vi "HOST_feedbacktest_datamonitoring_AAoptAOD_8-17-23.vi"() -> ()   [LabVIEW 2020]
uses:
  <vilib>/rvi/interface/nirviMethod/nirviMethod.xnode
  <vilib>/rvi/errors/niLvFpgaMergeErrorWithErrorCode.vi
  <instrlib>/_niInstr/Streaming/v1/Host/niInstr Streaming v1 Host.lvlib
  <vilib>/rvi/interface/nirviReadWriteControl/nirviReadWriteControl.xnode
  <vilib>/rvi/interface/nirviCloseFPGA/nirviCloseFPGA.xnode
  <vilib>/rvi/interface/nirviOpenFPGA/nirviOpenFPGA.xnode
  <vilib>/rvi/interface/Simulation/niFpgaSimulationCallBeginRW.vi
  <vilib>/rvi/errors/niLvFpgaAdjustHostInterfaceError.vi
  NiFpgaLv.dll
  <vilib>/Utility/error.llb/Error Cluster From Error Code.vi
  <vilib>/Utility/file.llb/Write Delimited Spreadsheet (string).vi
  <instrlib>/_niInstr/Streaming/v1/Host/Public/Start Finite Stream.vi
  <instrlib>/_niInstr/Streaming/v1/Host/Public/Wait for Stream.vi
  <vilib>/FPGAPlugInAG/Dynamic/niLvFpga_WriteFifo_Dynamic.vi
  <vilib>/FPGAPlugInAG/Dynamic/niLvFpga_Close_Dynamic.vi
  <vilib>/FPGAPlugInAG/Dynamic/niLvFpga_ReadFifo_Dynamic.vi
  <instrlib>/_niInstr/Streaming/v1/Host/Public/Start Continuous Stream.vi
  <vilib>/FPGAPlugInAG/Dynamic/niLvFpga_ConfigureFifo_Dynamic.vi
  <vilib>/FPGAPlugInAG/Dynamic/niLvFpga_StartFifo_Dynamic.vi
  FPGA Bitfiles/rfsignal_FPGATarget_feedbacktestdata_LKc-S6OmDz4.lvbitx
  <vilib>/FPGAPlugInAG/PXIe-7972R/niLvFpga_Open_PXIe-7972R.vi
  <vilib>/rvi/interface/common/dynamic/niFpgaDynamicAddResources.vi
  <vilib>/userdefined/Silver/nirio_resource_slv.ctl
  Controls/Clock Select.ctl
  PID/Typedef/niFpgaPID_ManualControl.ctl
  PID/Typedef/niFpgaPID_PIDGains.ctl
  PID/Typedef/niFpgaPID_OutputRange.ctl
  PID/Typedef/niFpgaPID_SetpointWeightings.ctl
  PID/Typedef/niFpgaPID_PIDActions.ctl
panel:
  out "actions":T1
  out "error":sgl
  out "output":sgl
  out "error 2":sgl
  out "error 3":sgl
  out "output 3":sgl
  out "actions 3":T1
  out "output 2":sgl
  out "actions 2":T1
  in  "Gains Z":T2[](array[typedef]) {"filter coefficient" min=0 max=1; "proportional gain" step=0.125}
  in  "setpoint weighting 3":T3={"proportional weighting (1)"=1.0, "derivative weighting (0)"=0.0} {"derivative weighting (0)" min=0 max=1; "proportional weighting (1)" min=0 max=1}
  in  "output range 3":T4={"output high (Inf)"=inf, "output low (-Inf)"=-inf}
  in  "manual control 3":T5
  in  "reset? (F) 3":bool
  in  "setpoint weighting 2":T3={"proportional weighting (1)"=1.0, "derivative weighting (0)"=0.0} {"derivative weighting (0)" min=0 max=1; "proportional weighting (1)" min=0 max=1}
  in  "output range 2":T4={"output high (Inf)"=inf, "output low (-Inf)"=-inf}
  in  "gains 2":T2 {"filter coefficient" min=0 max=1; "proportional gain" step=0.125}
  in  "manual control 2":T5
  in  "reset? (F) 2":bool
  in  "Feedback scaling z":fxp<+,16,4>
  in  "Feedback scaling x/y":fxp<+,16,4>
  in  "Apply feedback":bool
  in  "Data Trigger Level (V)":dbl
  in  "Record Size":u16=1024
  out "AI":waveform(dbl)[](graph)
  in  "Data Trigger When":enum8{"Trigger Above", "Trigger Below"}(ring)
  in  "Trigger Type":enum8{"Immediate", "Data Trigger", "TRIG input"}(ring)
  in  "Direction switch":bool
  in  "Step gain values":dbl
  in  "?":bool
  in  "% of max CH 1":dbl=85.0
  in  "% of max CH 0":dbl=85.0
  in  "setpoint weighting":T3={"proportional weighting (1)"=1.0, "derivative weighting (0)"=0.0} {"derivative weighting (0)" min=0 max=1; "proportional weighting (1)" min=0 max=1}
  in  "output range":T4={"output high (Inf)"=inf, "output low (-Inf)"=-inf}
  in  "gains":T2 {"filter coefficient" min=0 max=1; "proportional gain" step=0.125}
  in  "manual control":T5
  in  "reset? (F)":bool
  in  "write time ch0":bool
  in  "Record time for power sweep CH0":bool
  in  "Record time for power sweep CH1":bool
  in  "write time ch1":bool
  in  "save path for power calibration (dialog if empty)":path
  out "time check":u16=16
  in  "Cycles per step":u16=30
  in  "Gain Scan Endpoint (CH1)":dbl[](array[numeric])=[100.0, 100.0, 100.0, 100.0, 100.0, 100.0, 100.0, 100.0, 100.0, 100.0, 100.0, 100.0, 100.0, 100.0, 100.0, 100.0, 100.0, 100.0, 100.0, 100.0, 100.0, 100.0, 100.0, 100.0, 100.0, 100.0, 100.0, 100.0, 100.0, 100.0, 100.0, 100.0, 100.0, 100.0, 100.0, 100.0]
  in  "Gain Scan Endpoint (CH0)":dbl[](array[numeric])=[100.0, 100.0, 100.0, 100.0, 100.0, 100.0, 100.0, 100.0, 100.0, 100.0, 100.0, 100.0, 100.0, 100.0, 100.0, 100.0, 100.0, 100.0, 100.0, 100.0, 100.0, 100.0, 100.0, 100.0, 100.0, 100.0, 100.0, 100.0, 100.0, 100.0, 100.0, 100.0, 100.0, 100.0, 100.0, 100.0]
  in  "Scan End Setpoint (CH1)":dbl[](array[numeric])=[23.0, 24.0, 25.0, 26.0, 27.0, 28.0, 23.0, 24.0, 25.0, 26.0, 27.0, 28.0, 23.0, 24.0, 25.0, 26.0, 27.0, 28.0, 23.0, 24.0, 25.0, 26.0, 27.0, 28.0, 23.0, 24.0, 25.0, 26.0, 27.0, 28.0, 23.0, 24.0, 25.0, 26.0, 27.0, 28.0] format="%#_10f"
  in  "Scan CH1":bool
  in  "Scan CH0":bool
  in  "Fq Scan Endpoint (CH0)":dbl[](array[numeric])=[23.0, 23.0, 23.0, 23.0, 23.0, 23.0, 24.0, 24.0, 24.0, 24.0, 24.0, 24.0, 25.0, 25.0, 25.0, 25.0, 25.0, 25.0, 26.0, 26.0, 26.0, 26.0, 26.0, 26.0, 27.0, 27.0, 27.0, 27.0, 27.0, 27.0, 28.0, 28.0, 28.0, 28.0, 28.0, 28.0] format="%#_10f"
  in  "Refresh Integral":bool
  in  "Amp mod on/off":bool[](array[boolean])=[FALSE, FALSE, FALSE, FALSE, FALSE, FALSE, FALSE, FALSE, FALSE]
  in  "Mod Amp (%)":fxp<+,16,1>[](array[numeric])=[1.0, 1.0, 1.0, 1.0, 1.0, 1.0, 1.0, 1.0, 1.0]
  in  "Mod Fq (Hz) 3":dbl[](array[numeric])=[1.0, 1.0, 1.0, 1.0, 1.0, 1.0, 1.0, 1.0, 1.0] format="%#5.5f"
  in  "Wave 2 mod on/off":bool[](array[boolean])=[FALSE, FALSE, FALSE, FALSE, FALSE, FALSE, FALSE, FALSE, FALSE]
  in  "Mod strength (Hz) 2":dbl[](array[numeric])=[100000.0, 100000.0, 100000.0, 100000.0, 100000.0, 100000.0, 100000.0, 100000.0, 100000.0] format="%#_6p"
  in  "Mod Fq (Hz) 2":dbl[](array[numeric])=[1.0, 1.0, 1.0, 1.0, 1.0, 1.0, 1.0, 1.0, 1.0] format="%#5.5f"
  in  "Wave 1 mod on/off":bool[](array[boolean])=[FALSE, FALSE, FALSE, FALSE, FALSE, FALSE, FALSE, FALSE, FALSE]
  in  "Mod strength (Hz)":dbl[](array[numeric])=[100000.0, 100000.0, 100000.0, 100000.0, 100000.0, 100000.0, 100000.0, 100000.0, 100000.0] format="%#_6p"
  in  "Mod Time (Hz)":dbl[](array[numeric])=[1.0, 1.0, 1.0, 1.0, 1.0, 1.0, 1.0, 1.0, 1.0] format="%#5.5p"
  in  "Gain Scan Step Size % (CH1)":dbl=1.0
  in  "Gain Scan Step Size % (CH0)":dbl=1.0
  in  "Fq Scan Step Size MHz (CH1)":dbl=0.1
  in  "Fq Scan Step Size MHz (CH0)":dbl=0.1
  in  "Input pass through\nmode":enum16{"Wire", "Accum", "Accum-edge"}(ring)
  in  "# of beams":i8=36
  in  "Wave Reader CH 1 (MHz)":dbl[](array[numeric])=[23.0, 24.0, 25.0, 26.0, 27.0, 28.0, 23.0, 24.0, 25.0, 26.0, 27.0, 28.0, 23.0, 24.0, 25.0, 26.0, 27.0, 28.0, 23.0, 24.0, 25.0, 26.0, 27.0, 28.0, 23.0, 24.0, 25.0, 26.0, 27.0, 28.0, 23.0, 24.0, 25.0, 26.0, 27.0, 28.0] format="%#_15f"
  in  "Gain CH 1 (%)":dbl[](array[numeric])=[100.0, 100.0, 100.0, 100.0, 100.0, 100.0, 100.0, 100.0, 100.0, 100.0, 100.0, 100.0, 100.0, 100.0, 100.0, 100.0, 100.0, 100.0, 100.0, 100.0, 100.0, 100.0, 100.0, 100.0, 100.0, 100.0, 100.0, 100.0, 100.0, 100.0, 100.0, 100.0, 100.0, 100.0, 100.0, 100.0]
  in  "Remove transition edges":i32=5
  in  "Time per beam in us":i32=20
  in  "stop":bool
  in  "Gain CH 0 (%)":dbl[](array[numeric])=[100.0, 100.0, 100.0, 100.0, 100.0, 100.0, 100.0, 100.0, 100.0, 100.0, 100.0, 100.0, 100.0, 100.0, 100.0, 100.0, 100.0, 100.0, 100.0, 100.0, 100.0, 100.0, 100.0, 100.0, 100.0, 100.0, 100.0, 100.0, 100.0, 100.0, 100.0, 100.0, 100.0, 100.0, 100.0, 100.0]
  in  "Wave Reader CH 0 (MHz)":dbl[](array[numeric])=[23.0, 23.0, 23.0, 23.0, 23.0, 23.0, 24.0, 24.0, 24.0, 24.0, 24.0, 24.0, 25.0, 25.0, 25.0, 25.0, 25.0, 25.0, 26.0, 26.0, 26.0, 26.0, 26.0, 26.0, 27.0, 27.0, 27.0, 27.0, 27.0, 27.0, 28.0, 28.0, 28.0, 28.0, 28.0, 28.0] format="%#_13f"
  in  "Magnitude Initialization Vpp":dbl[](array[numeric])=[1.0, 1.0] format="%0.2p"
  in  "Frequencies (Hz)":dbl[](array[numeric])=[10000.0, 10000.0] format="%5.0p"
  in  "Signal Type":T6(ring)
  in  "Sampling Info":cluster{"Fs":dbl, "#s":dbl}={"Fs"=163840000.0, "#s"=65536.0} {"Fs" format="%#_5p"}
  out "Error Out":errorcluster
  in  "Update Waveform":bool
  in  "Clock Select":T7 items=["Internal Clock", "Internal Clock w/ Ref via CLK/REF IN", "Internal Clock w/ Ref via Sync Clock", "External Clock via CLK/REF IN"]
  in  "Rate of External Sample Clock (MHz)":u16=100 min=60 max=100 step=1
  in  "RIO Resource":T8="RIO0"
  # "General Feedback Settings"
  # "Time cycle loop processing"
  # "Shared Feedback Controls"
  # "Don't change"
  # "Waveform Initialization"
  # "Modulation disabled for now while testing FPGA code, too high compiling time for quick turn around"
  # "Controls the Output of the FPGA\nEach row corresponds to one beam created by the AOD\nCH 0 is Output 0 on the FPGA card and controls the () direction on the AOD; CH 1 is Output 1 on the FPGA card and controls the () direction on the AOD\n\nThe  set frequency is the output of the FPGA, this is then mixed with a 50MHz LO to be in the AOD's bandwidth of 75 +- 15MHz\n\nThe gain is the percentage of the 1Vpp initialized voltage to output. It is in percentage and goes from 0 - 100\n\nIt will play the first n rows of tones, \nwhere n is the \"# of beams\" value."
  # "DO NOT CHANGE"
  # "X Feedback"
  # "These allow you to smoothly ramp between frequencies or gain settings for each individual beam.\nThe channels scan independently, but it will simultaneously ramp every fq/gain in the channel to their desired point.\nThey should update to match the main control setting when scanning is not enabled."
  # "Ch 0 Wave Sin Modulation"
  # "Ch 1 Wave Sin Modulation"
  # "Amplitude Sin Modulation"
  # "Do not change these values while waiting for scan"
  # "Main control for the tones played on FPGA analog out 0\nSets the base, static frequency to play"
  # "Main control for the tones played on FPGA analog out 1\nSets the base, static frequency to play"
  # "Ch 0 Output Waveforms"
  # "Ch 1 Output Waveforms"
  # "Y Feedback"
  # "Ch0"
  # "Ch1"
  # "Modulates the output frequencies of CH 0 in a sine wave pattern\n\nMod time: Sets how fast the modulation goes\n     (e.g. 1 Hz means it will go through a full cycle in 1 second)\n\nMod strength: Sets the amplitude of the modulation\n     (e.g. 100kHz means that the frequency will go between \n      set frequency + 100kHz and set frequency - 100kHz)"
  # "Modulates the output frequencies of CH 1 in a sine wave pattern\n\nMod time: Sets how fast the modulation goes\n     (e.g. 1 Hz means it will go through a full cycle in 1 second)\n\nMod strength: Sets the amplitude of the modulation\n     (e.g. 100kHz means that the frequency will go between \n      set frequency + 100kHz and set frequency - 100kHz)"
  # "Modulates the output amplitude of CH 0 in a sine wave pattern\n\nMod time: Sets how fast the modulation goes\n     (e.g. 1 Hz means it will go through a full cycle in 1 second)\n\nMod strength: Sets the amplitude of the modulation\n     (e.g. 5% means that the amplitude will go between \n      set amp + 5%  and set amp  - 5%)"
  # "Z\nFeedback"
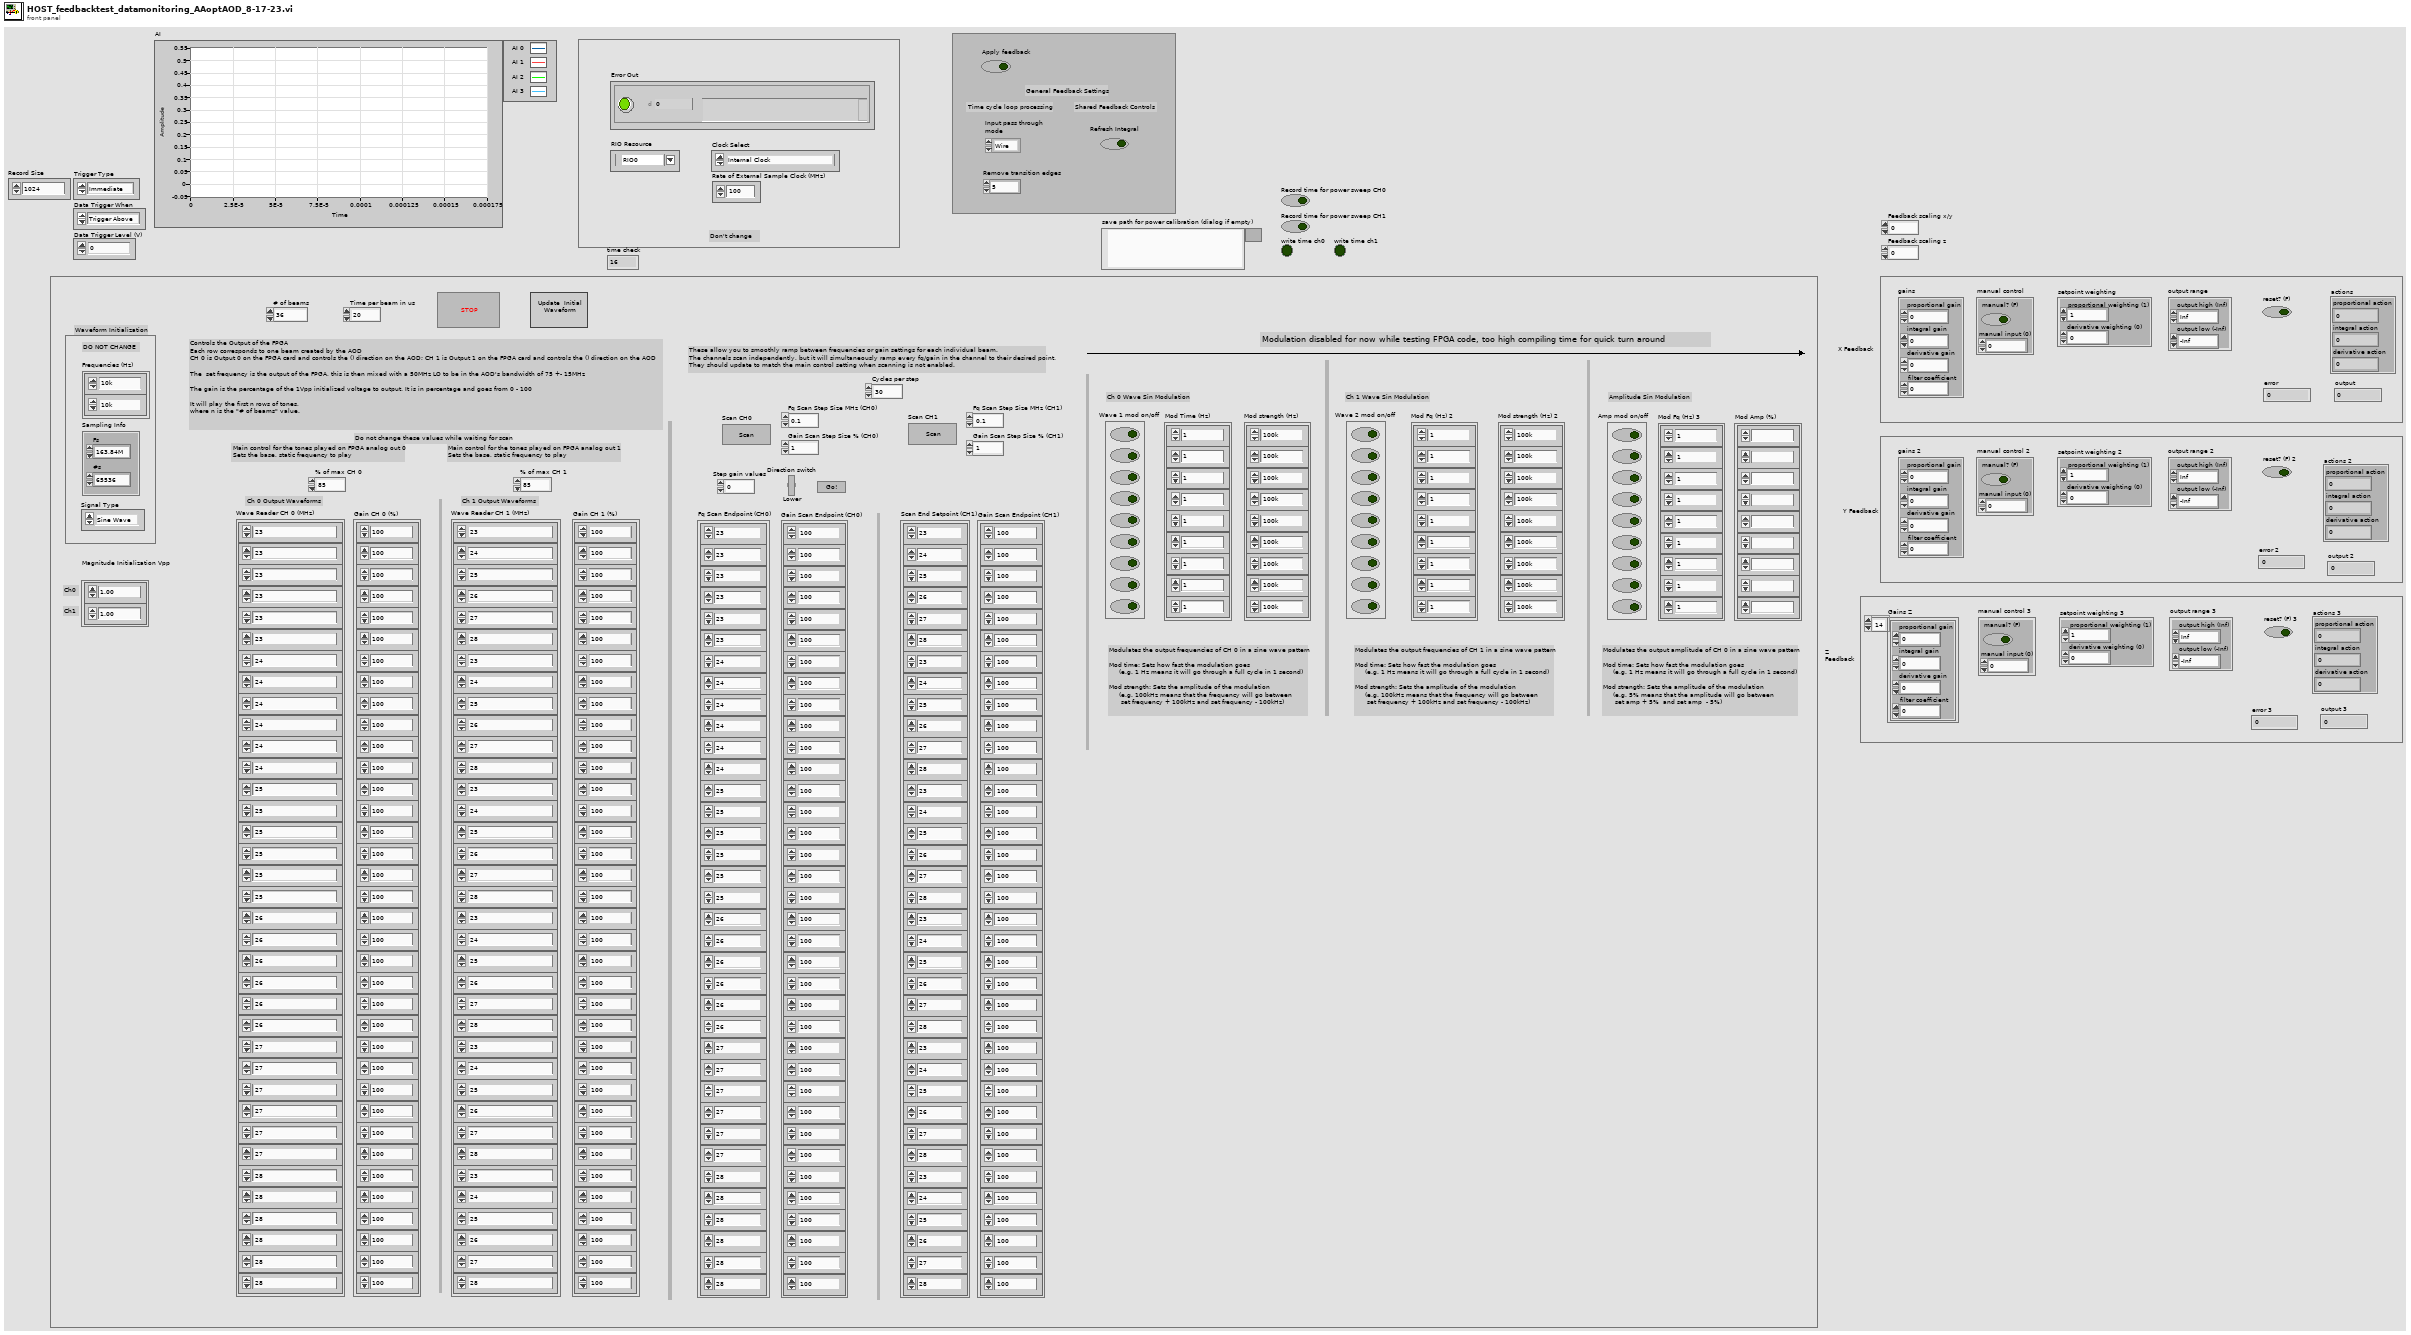
[diagram p1: front panel]
types:
  T1 = typedef "niFpgaPID_PIDActions.ctl" = cluster{"proportional action":sgl, "integral action":sgl, "derivative action":sgl}
  T2 = typedef "niFpgaPID_PIDGains.ctl" = cluster{"proportional gain":sgl, "integral gain":sgl, "derivative gain":sgl, "filter coefficient":sgl}
  T3 = typedef "niFpgaPID_SetpointWeightings.ctl" = cluster{"proportional weighting (1)":sgl, "derivative weighting (0)":sgl}
  T4 = typedef "niFpgaPID_OutputRange.ctl" = cluster{"output high (Inf)":sgl, "output low (-Inf)":sgl}
  T5 = typedef "niFpgaPID_ManualControl.ctl" = cluster{"manual? (F)":bool, "manual input (0)":sgl}
  T6 = enum16{"Sine Wave", "Triangle Wave", "Square Wave", "Sawtooth Wave"}
  T7 = typedef "Clock Select.ctl" = u16
  T8 = typedef "nirio_resource_slv.ctl" = tag
  T9 = cluster{"proportional action":sgl, "integral action":sgl, "derivative action":sgl}
  T10 = cluster{"level":i16, "trigger when":enum8{"Trigger Above", "Trigger Below"}}
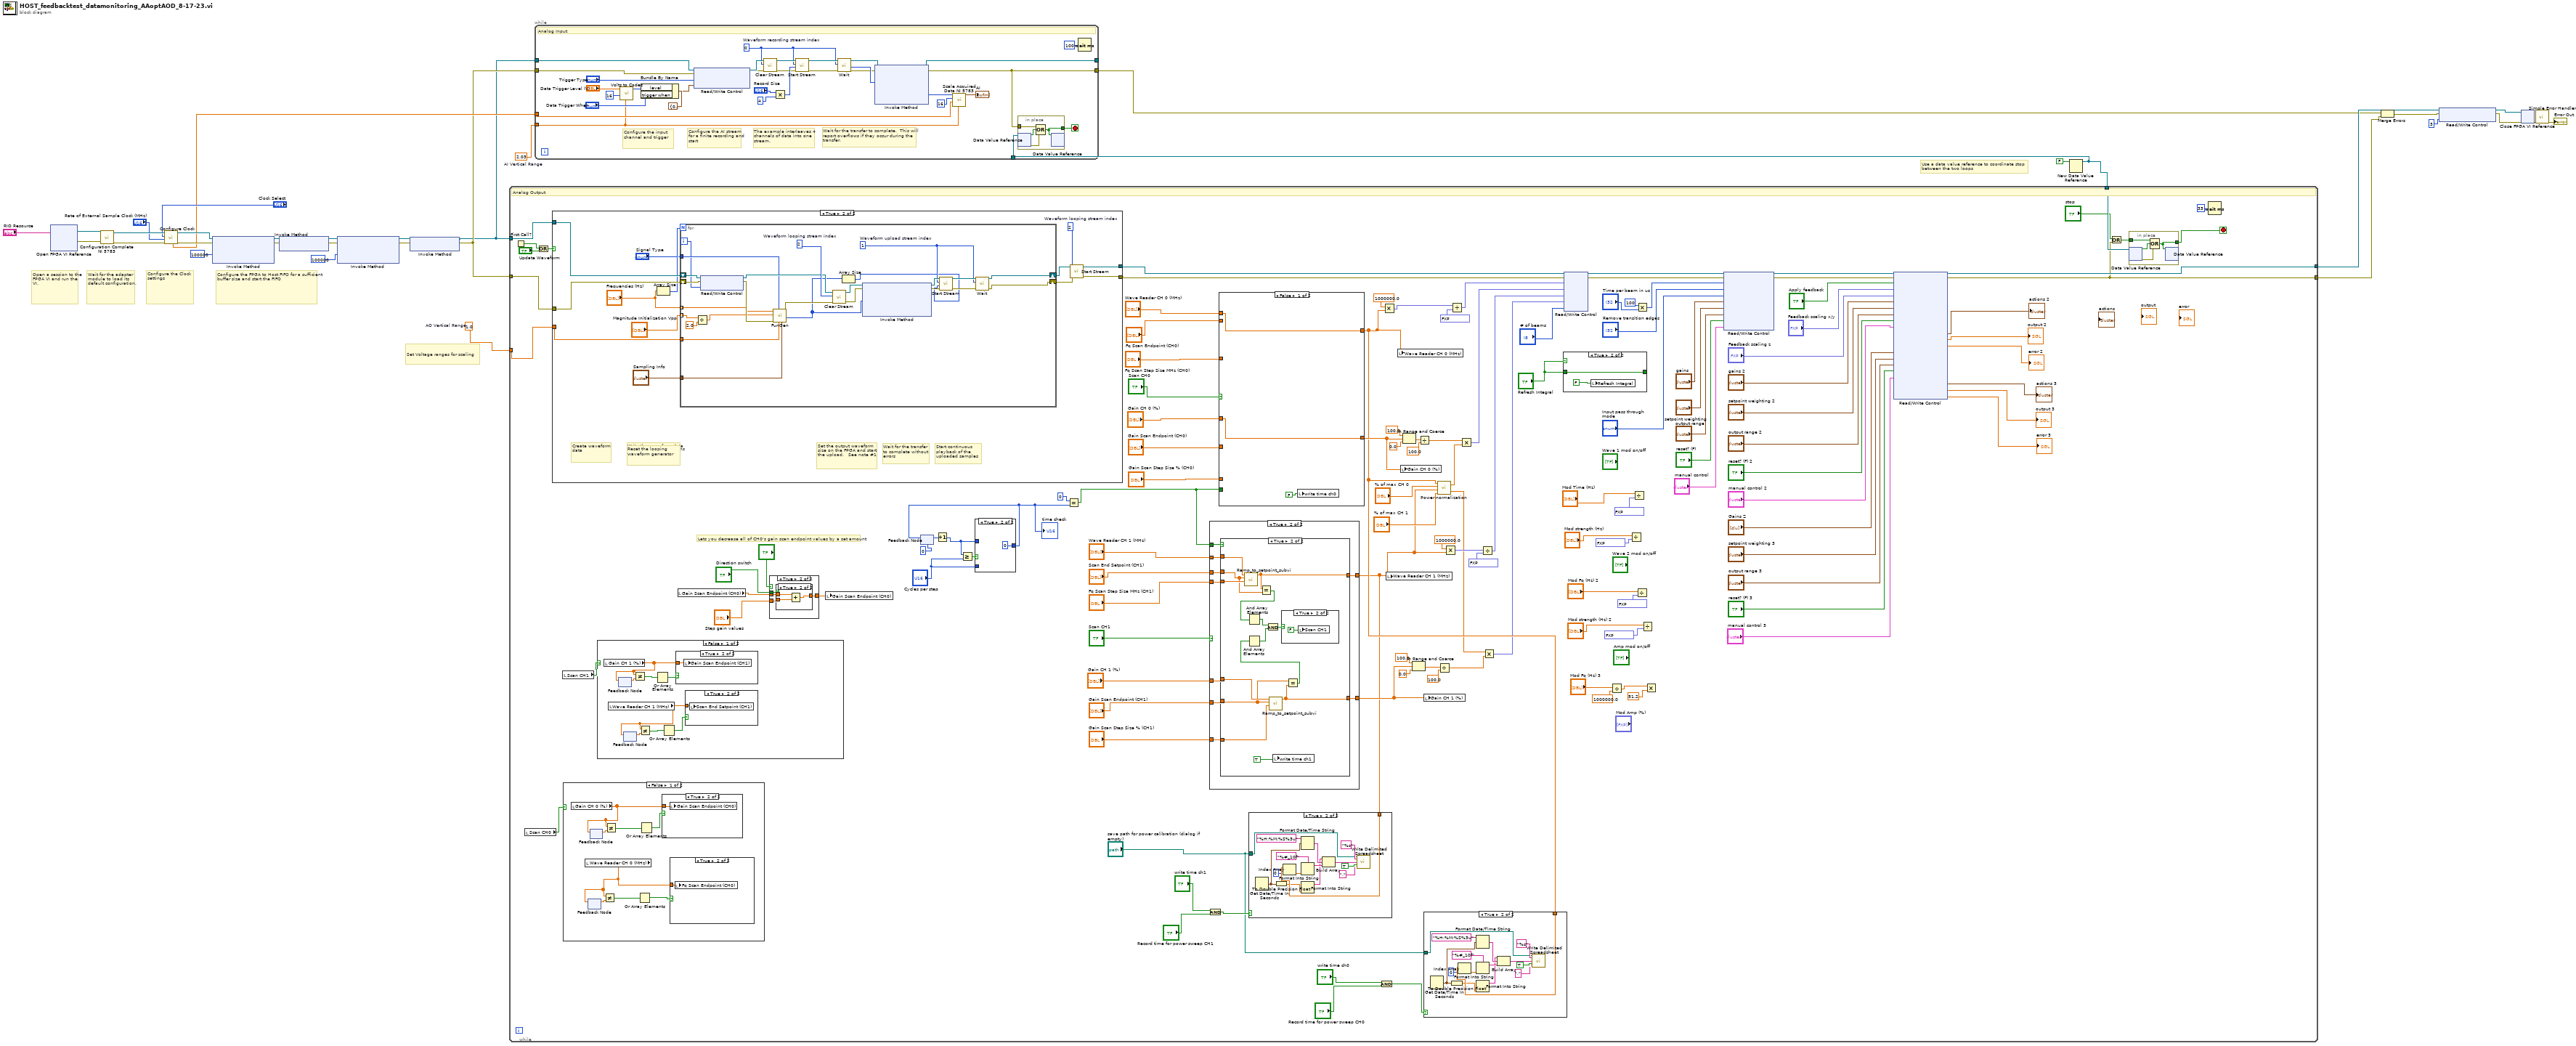
[diagram p0: block diagram]
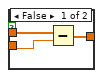
[diagram p3: hidden frame]
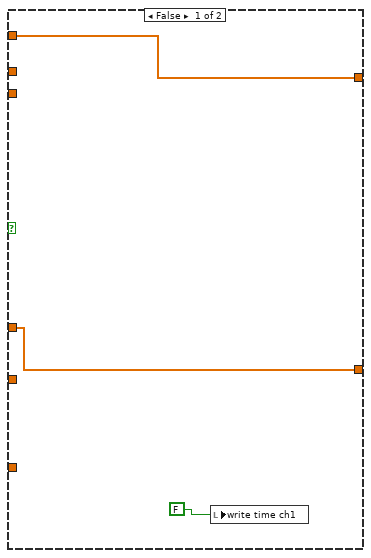
[diagram p6: hidden frame]
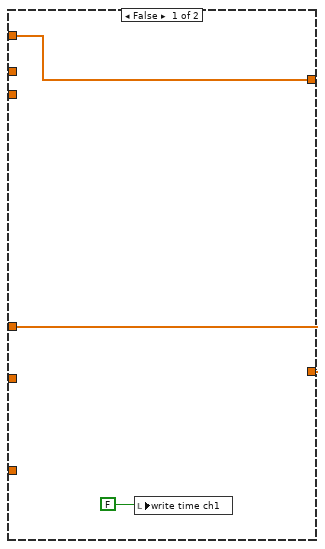
[diagram p7: hidden frame]
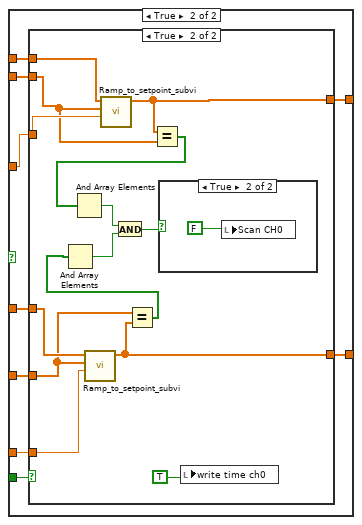
[diagram p9: hidden frame]
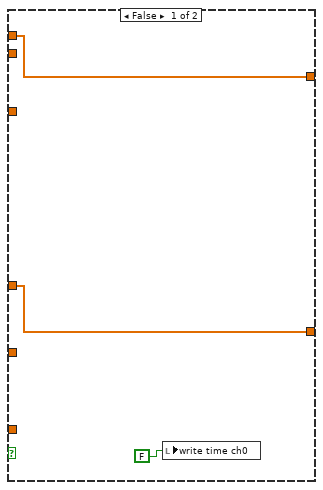
[diagram p10: hidden frame]
diagram:
  w13 = 2.03  # AI Vertical Range
  w21 = 1.0  # AO Vertical Range
  # "Use a data value reference to coordinate stop between the two loops"
  # "Set Voltage ranges for scaling"
  # "Configure the Clock settings"
  # "Configure the FPGA to Host FIFO for a sufficient buffer size and start the FIFO"
  # "Wait for the adapter module to load its default configuration."
  # "Open a session to the FPGA VI and run the VI."
  n1 = xnode "Open FPGA VI Reference"("resource name"="RIO Resource") -> ("FPGA VI Reference Out"=w19:refnum<k20>, "error out"=w18:errorcluster)  [unwired: 1 in]
  n2 = call "Configuration Complete NI 5783.vi"("error in"=w18, "FPGA VI Reference In"=w19) -> ("error out"=w29:errorcluster, "FPGA VI Reference Out"=w30:refnum<k20>)  [unwired: 7 in, 1 out]
  n3 = call "Configure Clock.vi"("error in (no error)"=w29, "Rate of External Sample Clock (MHz)"="Rate of External Sample Clock (MHz)", "Clock Select"="Clock Select", "FPGA VI Reference In"=w30) -> ("error out"=w27:errorcluster, "FPGA VI Reference Out"=w28:refnum<k20>, "Sampling Rate"=w12:dbl)  [unwired: 3 in, 2 out]
  n4 = xnode "Invoke Method"("FPGA VI Reference In"=w28, "error in"=w27, "Requested Depth"=u32 100000) -> ("FPGA VI Reference Out"=w33:refnum<k20>, "error out"=w32:errorcluster)  [unwired: 1 out]
  n5 = xnode "Invoke Method"("FPGA VI Reference In"=w33, "error in"=w32) -> ("FPGA VI Reference Out"=w4:refnum<k20>, "error out"=w7:errorcluster)
  n6 = xnode "Invoke Method"("FPGA VI Reference In"=w4, "error in"=w7, "Requested Depth"=u32 100000) -> ("FPGA VI Reference Out"=w3:refnum<k20>, "error out"=w6:errorcluster)  [unwired: 1 out]
  n7 = xnode "Invoke Method"("FPGA VI Reference In"=w3, "error in"=w6) -> ("FPGA VI Reference Out"=w2:refnum<k20>, "error out"=w5:errorcluster)
  n8 = New Data Value Reference(data value=FALSE ("Stopped")) -> (data value reference=w10:refnum<data-value>)  [unwired: 1 in, 1 out]
  n9 = while {
    tunnel: w5 -> [w153]
    tunnel: w2 -> [w159]
    tunnel: [w54] -> w17
    tunnel: w10 -> [w154]
    tunnel: w21 -> [w152]
    tunnel: [w52] -> w8
    stop <- w59 stop-if-true
    # "Lets you decrease all of CH0's gain scan endpoint values by a set amount"
    # "Analog Output"
    n10 = First Call?() -> (First Call?: T/F=w155:bool)
    n11 = local read "Scan CH0"() -> (w102:bool)
    n12 = Or(x=w155, y="Update Waveform") -> (x .or. y?=w156:bool)
    n13 = case shown="True" w156 {
      tunnel: [w291 w304] -> w151
      tunnel: [w290 w303] -> w150
      tunnel: w159 -> [w291 w301]
      tunnel: w153 -> [w290 w300]
      tunnel: w152 -> [_ w302]
      frame False {
      }
      frame True {
        w299 = 2  # Waveform looping stream index
        # "Loop over the waveforms to combine"
        # "Reset the looping waveform generator"
        # "Start continuous playback of the uploaded samples"
        # "Wait for the transfer to complete without errors"
        # "Set the output waveform size on the FPGA and start the upload.   See note #1"
        # "Write the waveform data to the FPGA for generation"
        # "Create waveform data"
        n14 = Array Size(array="Frequencies (Hz)") -> (size(s)=w294:i32)
        n15 = for {
          N: w294 -> [_]
          tunnel: w302 -> [w319]
          shift-right: [w313] -> w298
          shift-left: w301 -> [w318]
          shift-right: [w312] -> w297
          shift-left: w300 -> [w316]
          tunnel: "Frequencies (Hz)" -> [w311] mode=indexing
          tunnel: "Magnitude Initialization Vpp" -> [w307] mode=indexing
          tunnel: "Sampling Info" -> [w310]
          tunnel: "Signal Type" -> [w309]
          i -> [w308]
          w320 = 2  # Waveform looping stream index
          w325 = 1  # Waveform upload stream index
          n16 = Divide(x=w307, y=2.0) -> (x/y=w306:dbl)
          n17 = xnode "Read/Write Control"("FPGA VI Reference In"=w318, "error in"=w316, "Upload selector"=w308) -> ("FPGA VI Reference Out"=w317:refnum<k20>, "error out"=w315:errorcluster)
          n18 = call "FunGen.vi"("sampling info"=w310, "range (Vpp)"=w319, "signal type"=w309, "error in (no error)"=w315, "amplitude"=w306, "frequency"=w311) -> ("error out"=w321:errorcluster, "Waveform Data"=w314:i16[])  [unwired: 2 in, 2 out]
          n19 = call <instrlib>:"Clear Stream.vi"("error in (no error)"=w321, "stream index"=w320, "refnum in"=w317) -> ("error out"=w323:errorcluster, "refnum out"=w324:refnum<k20>)  [unwired: 7 in]
          n20 = Array Size(array=w314) -> (size(s)=w322:i32)
          n21 = xnode "Invoke Method"("FPGA VI Reference In"=w324, "error in"=w323, "Data"=w314) -> ("FPGA VI Reference Out"=w329:refnum<k20>, "error out"=w328:errorcluster)  [unwired: 1 in, 1 out]
          n22 = call-poly <instrlib>:"Start Stream.vi"("error in (no error)"=w328, "num samples"=w322, "stream index"=w325, "refnum in"=w329) -> ("error out"=w326:errorcluster, "refnum out"=w327:refnum<k20>)  [unwired: 6 in]
          n23 = call-poly <instrlib>:"Wait.vi"("error in (no error)"=w326, "stream index"=w325, "refnum in"=w327) -> ("error out"=w312:errorcluster, "refnum out"=w313:refnum<k20>)  [unwired: 5 in, 2 out]
        }
        n24 = call-poly <instrlib>:"Start Stream.vi"("error in (no error)"=w297, "stream index"=w299, "refnum in"=w298) -> ("error out"=w303:errorcluster, "refnum out"=w304:refnum<k20>)  [unwired: 7 in]
      }
    }
    n25 = local read "Scan CH1"() -> (w103:bool)
    n26 = case shown="False" w102 {
      frame False {
        n27 = local read "Gain CH 0 (%)"() -> (w263:dbl[])
        n28 = local read "Wave Reader CH 0 (MHz)"() -> (w270:dbl[])
        n29 = feedback-in #1(w270) -> ()
        n30 = feedback #1() -> (w269:dbl[])  [unwired: 1 in]
        n31 = feedback #2() -> (w266:dbl[])  [unwired: 1 in]
        n32 = feedback-in #2(w263) -> ()
        n33 = Not Equal?(x=w270, y=w269) -> (x != y?=w268:bool[])
        n34 = Not Equal?(x=w263, y=w266) -> (x != y?=w265:bool[])
        n35 = Or Array Elements(Boolean array=w268) -> (logical OR=w267:bool)
        n36 = Or Array Elements(Boolean array=w265) -> (logical OR=w264:bool)
        n37 = case shown="True" w264 {
          tunnel: w263 -> [_ w271]
          frame False {
          }
          frame True {
            n38 = local write "Gain Scan Endpoint (CH0)"(w271) -> ()
          }
        }
        n39 = case shown="True" w267 {
          tunnel: w270 -> [_ w272]
          frame False {
          }
          frame True {
            n40 = local write "Fq Scan Endpoint (CH0)"(w272) -> ()
          }
        }
      }
      frame True {
      }
    }
    n41 = case shown="False" w103 {
      frame False {
        n42 = local read "Gain CH 1 (%)"() -> (w273:dbl[])
        n43 = local read "Wave Reader CH 1 (MHz)"() -> (w277:dbl[])
        n44 = feedback #3() -> (w276:dbl[])  [unwired: 1 in]
        n45 = feedback-in #3(w273) -> ()
        n46 = feedback #4() -> (w280:dbl[])  [unwired: 1 in]
        n47 = feedback-in #4(w277) -> ()
        n48 = Not Equal?(x=w273, y=w276) -> (x != y?=w275:bool[])
        n49 = Not Equal?(x=w277, y=w280) -> (x != y?=w279:bool[])
        n50 = Or Array Elements(Boolean array=w275) -> (logical OR=w274:bool)
        n51 = Or Array Elements(Boolean array=w279) -> (logical OR=w278:bool)
        n52 = case shown="True" w274 {
          tunnel: w273 -> [_ w281]
          frame False {
          }
          frame True {
            n53 = local write "Gain Scan Endpoint (CH1)"(w281) -> ()
          }
        }
        n54 = case shown="True" w278 {
          tunnel: w277 -> [_ w282]
          frame False {
          }
          frame True {
            n55 = local write "Scan End Setpoint (CH1)"(w282) -> ()
          }
        }
      }
      frame True {
      }
    }
    n56 = local read "Gain Scan Endpoint (CH0)"() -> (w61:dbl[])
    n57 = case shown="True" "?" {
      tunnel: w61 -> [w160 w163]
      tunnel: [w160 w164] -> w62
      tunnel: "Step gain values" -> [_ w162]
      tunnel: "Direction switch" -> [_ w161]
      frame False {
      }
      frame True {
        n58 = case shown="True" w161 {
          tunnel: [w167 w169] -> w164
          tunnel: w163 -> [w166 w168]
          tunnel: w162 -> [w165 w170]
          frame False {
            n59 = Subtract(x=w166, y=w165) -> (x-y=w167:dbl[])
          }
          frame True {
            n60 = Add(x=w168, y=w170) -> (x+y=w169:dbl[])
          }
        }
      }
    }
    n61 = local write "Gain Scan Endpoint (CH0)"(w62) -> ()
    n62 = feedback #5(u16 0) -> (w98:u16)
    n63 = Increment(x=w98) -> (x+1=w96:u16)
    n64 = Greater Or Equal?(x=w96, y="Cycles per step") -> (x >= y?=w97:bool)
    n65 = case shown="True" w97 {
      tunnel: w96 -> [w261 _]
      tunnel: "Cycles per step" -> [_ _]
      tunnel: [w261 u16 0] -> w91
      frame False {
      }
      frame True {
      }
    }
    "time check" <- w91
    n66 = feedback-in #5(w91) -> ()
    n67 = Equal?(x=u16 0, y=w91) -> (x = y?=w92:bool)
    n68 = And(x="write time ch1", y="Record time for power sweep CH1") -> (x .and. y?=w90:bool)
    n69 = case shown="True" "Scan CH1" {
      tunnel: "Fq Scan Step Size MHz (CH1)" -> [_ w212]
      tunnel: [w203 w211] -> w70
      tunnel: "Wave Reader CH 1 (MHz)" -> [w203 w210]
      tunnel: "Scan End Setpoint (CH1)" -> [_ w209]
      tunnel: "Gain Scan Step Size % (CH1)" -> [_ w208]
      tunnel: "Gain CH 1 (%)" -> [w202 w207]
      tunnel: "Gain Scan Endpoint (CH1)" -> [_ w206]
      tunnel: [w202 w205] -> w104
      tunnel: w92 -> [_ w204]
      frame False {
        n70 = local write "write time ch1"(FALSE) -> ()
      }
      frame True {
        n71 = case shown="True" w204 {
          tunnel: w210 -> [w215 w229]
          tunnel: w209 -> [_ w227]
          tunnel: w212 -> [_ w228]
          tunnel: [w215 w226] -> w211
          tunnel: w207 -> [w214 w224]
          tunnel: w206 -> [_ w223]
          tunnel: w208 -> [_ w222]
          tunnel: [w214 w217] -> w205
          frame False {
            n72 = local write "write time ch1"(FALSE) -> ()
          }
          frame True {
            n73 = call "Ramp_to_setpoint_subvi.vi"("Numeric"=w228, "Scan to Fq (CH0)"=w227, "Wave Reader CH 0 (Y)"=w229) -> ("Array"=w226:dbl[])  [unwired: 8 in]
            n74 = Equal?(x=w226, y=w227) -> (x = y?=w225:bool[])
            n75 = And Array Elements(Boolean array=w225) -> (logical AND=w219:bool)
            n76 = call "Ramp_to_setpoint_subvi.vi"("Numeric"=w222, "Scan to Fq (CH0)"=w223, "Wave Reader CH 0 (Y)"=w224) -> ("Array"=w217:dbl[])  [unwired: 8 in]
            n77 = local write "write time ch1"(TRUE) -> ()
            n78 = Equal?(x=w223, y=w217) -> (x = y?=w218:bool[])
            n79 = And Array Elements(Boolean array=w218) -> (logical AND=w220:bool)
            n80 = And(x=w219, y=w220) -> (x .and. y?=w221:bool)
            n81 = case shown="True" w221 {
              frame False {
              }
              frame True {
                n82 = local write "Scan CH1"(FALSE) -> ()
              }
            }
          }
        }
      }
    }
    n83 = case shown="False" "Scan CH0" {
      tunnel: "Fq Scan Step Size MHz (CH0)" -> [_ w242]
      tunnel: "Wave Reader CH 0 (MHz)" -> [w233 w241]
      tunnel: "Fq Scan Endpoint (CH0)" -> [_ w240]
      tunnel: [w233 w239] -> w71
      tunnel: "Gain CH 0 (%)" -> [w232 w238]
      tunnel: "Gain Scan Endpoint (CH0)" -> [_ w237]
      tunnel: [w232 w236] -> w112
      tunnel: "Gain Scan Step Size % (CH0)" -> [_ w235]
      tunnel: w92 -> [_ w234]
      frame False {
        n84 = local write "write time ch0"(FALSE) -> ()
      }
      frame True {
        n85 = case shown="True" w234 {
          tunnel: w241 -> [w245 w259]
          tunnel: w240 -> [_ w257]
          tunnel: w242 -> [_ w258]
          tunnel: [w245 w256] -> w239
          tunnel: w238 -> [w244 w254]
          tunnel: w237 -> [_ w251]
          tunnel: w235 -> [_ w253]
          tunnel: [w244 w252] -> w236
          frame False {
            n86 = local write "write time ch0"(FALSE) -> ()
          }
          frame True {
            n87 = call "Ramp_to_setpoint_subvi.vi"("Numeric"=w253, "Scan to Fq (CH0)"=w251, "Wave Reader CH 0 (Y)"=w254) -> ("Array"=w252:dbl[])  [unwired: 8 in]
            n88 = call "Ramp_to_setpoint_subvi.vi"("Numeric"=w258, "Scan to Fq (CH0)"=w257, "Wave Reader CH 0 (Y)"=w259) -> ("Array"=w256:dbl[])  [unwired: 8 in]
            n89 = Equal?(x=w251, y=w252) -> (x = y?=w250:bool[])
            n90 = And Array Elements(Boolean array=w250) -> (logical AND=w247:bool)
            n91 = Equal?(x=w256, y=w257) -> (x = y?=w255:bool[])
            n92 = And Array Elements(Boolean array=w255) -> (logical AND=w248:bool)
            n93 = And(x=w248, y=w247) -> (x .and. y?=w249:bool)
            n94 = case shown="True" w249 {
              frame False {
              }
              frame True {
                n95 = local write "Scan CH0"(FALSE) -> ()
              }
            }
            n96 = local write "write time ch0"(TRUE) -> ()
          }
        }
      }
    }
    n97 = case shown="True" w90 {
      tunnel: w70 -> [_ w193]
      tunnel: "save path for power calibration (dialog if empty)" -> [_ w186]
      frame False {
      }
      frame True {
        n98 = Get Date/Time In Seconds() -> (seconds since 1Jan1904=w189:timestamp)
        n99 = To Double Precision Float(number=w189) -> (double precision float=w188:dbl)
        n100 = Index Array(array=w193, index=0) -> (element=w191:dbl)
        n101 = Format Date/Time String(time format string (%c)="%H:%M:%S%3u", seconds (now)=w189) -> (date/time string=w196:string)  [unwired: 1 in]
        n102 = Format Into String(format string="%#_10f", w191) -> (resulting string=w195:string)  [unwired: 2 in, 1 out]
        n103 = Format Into String(w188) -> (resulting string=w187:string)  [unwired: 3 in, 1 out]
        n104 = Build Array(w187, w196, w195) -> (w190:string[])
        n105 = call-poly <vilib>:"Write Delimited Spreadsheet.vi"("file path (dialog if empty)"=w186, "format (%s)"="%s" ("format (%.3f)"), "1D data"=w190, "append to file? (new file:F)"=TRUE, "delimiter (\\t)"="," ("delimiter (\\t)")) -> ()  [unwired: 9 in, 2 out]
      }
    }
    n106 = And(x="write time ch0", y="Record time for power sweep CH0") -> (x .and. y?=w86:bool)
    n107 = Multiply(x=1000000.0, y=w71) -> (x*y=w124:fxp<+/-,64,32>[])
    n108 = local write "Wave Reader CH 1 (MHz)"(w70) -> ()
    n109 = local write "Wave Reader CH 0 (MHz)"(w71) -> ()
    n110 = local write "Gain CH 0 (%)"(w112) -> ()
    n111 = In Range and Coerce(upper limit=100.0, x=w112, lower limit=0.0) -> (coerced(x)=w115:dbl[])  [unwired: 1 out]
    n112 = In Range and Coerce(upper limit=100.0, x=w104, lower limit=0.0) -> (coerced(x)=w110:dbl[])  [unwired: 1 out]
    n113 = Divide(x=w115, y=100.0) -> (x/y=w75:dbl[])
    n114 = local write "Gain CH 1 (%)"(w104) -> ()
    n115 = case shown="True" w86 {
      tunnel: w71 -> [_ w178]
      tunnel: "save path for power calibration (dialog if empty)" -> [_ w171]
      frame False {
      }
      frame True {
        n116 = Get Date/Time In Seconds() -> (seconds since 1Jan1904=w174:timestamp)
        n117 = To Double Precision Float(number=w174) -> (double precision float=w173:dbl)
        n118 = Index Array(array=w178, index=0) -> (element=w176:dbl)
        n119 = Format Date/Time String(time format string (%c)="%H:%M:%S%3u", seconds (now)=w174) -> (date/time string=w181:string)  [unwired: 1 in]
        n120 = Format Into String(format string="%#_10f", w176) -> (resulting string=w180:string)  [unwired: 2 in, 1 out]
        n121 = Format Into String(w173) -> (resulting string=w172:string)  [unwired: 3 in, 1 out]
        n122 = Build Array(w172, w181, w180) -> (w175:string[])
        n123 = call-poly <vilib>:"Write Delimited Spreadsheet.vi"("file path (dialog if empty)"=w171, "format (%s)"="%s" ("format (%.3f)"), "1D data"=w175, "append to file? (new file:F)"=TRUE, "delimiter (\\t)"="," ("delimiter (\\t)")) -> ()  [unwired: 9 in, 2 out]
      }
    }
    n124 = call "Power normalization.vi"("% of max CH 1"="% of max CH 1", "CH 1 frequency"=w70, "% of max CH 0"="% of max CH 0", "CH 0 frequency"=w71) -> ("Normalized CH1"=w67:dbl[], "Normalized CH 0"=w72:dbl[])
    n125 = Divide(x=w110, y=100.0) -> (x/y=w68:dbl[])
    n126 = Multiply(x=1000000.0, y=w70) -> (x*y=w121:fxp<+/-,64,32>[])
    n127 = Divide(x=w124, y=fxp<+,32,16> 6103.515625) -> (x/y=w83:fxp<+,33,16>[])
    n128 = Multiply(x=w75, y=w72) -> (x*y=w76:fxp<+,32,4>[])
    n129 = Divide(x=w121, y=fxp<+,32,16> 6103.515625) -> (x/y=w82:fxp<+,33,16>[])
    n130 = Multiply(x=w67, y=w68) -> (x*y=w69:fxp<+,32,4>[])
    n131 = case shown="True" "Refresh Integral" {
      tunnel: [w283 w284] -> _
      tunnel: "Refresh Integral" -> [w283 w284]
      frame False {
      }
      frame True {
        n132 = local write "Refresh Integral"(FALSE) -> ()
      }
    }
    n133 = xnode "Read/Write Control"("FPGA VI Reference In"=w151, "error in"=w150, "Wave 1"=w83, "Amp 1"=w76, "Wave 2"=w82, "Amp 2"=w69, "Size"="# of beams") -> ("FPGA VI Reference Out"=w148:refnum<k20>, "error out"=w147:errorcluster)
    n134 = Divide(x="Mod Fq (Hz) 3", y=1000000.0) -> (x/y=w135:dbl[])
    n135 = Divide(x="Mod strength (Hz)", y=fxp<+,32,16> 6103.515625) -> ()  [unwired: 1 out]
    n136 = Divide(x="Mod Time (Hz)", y=fxp<+,32,16> 6103.515625) -> ()  [unwired: 1 out]
    n137 = Divide(x="Mod Fq (Hz) 2", y=fxp<+,32,16> 6103.515625) -> ()  [unwired: 1 out]
    n138 = Multiply(x=100, y="Time per beam in us") -> (x*y=w144:i32)
    n139 = Divide(x="Mod strength (Hz) 2", y=fxp<+,32,16> 6103.515625) -> ()  [unwired: 1 out]
    n140 = Multiply(x=w135, y=51.2) -> ()  [unwired: 1 out]
    n141 = xnode "Read/Write Control"("FPGA VI Reference In"=w148, "error in"=w147, "Timeshare"=w144, "Edge size"="Remove transition edges", "Pass selector"="Input pass through\nmode", "gains"="gains", "setpoint weighting"="setpoint weighting", "output range"="output range", "reset? (F)"="reset? (F)", "manual control"="manual control") -> ("FPGA VI Reference Out"=w55:refnum<k20>, "error out"=w56:errorcluster)
    n142 = xnode "Read/Write Control"("FPGA VI Reference In"=w55, "error in"=w56, "Apply feedback"="Apply feedback", "Feedback scaling x/y"="Feedback scaling x/y", "Feedback scaling z"="Feedback scaling z", "gains 2"="gains 2", "setpoint weighting 2"="setpoint weighting 2", "output range 2"="output range 2", "reset? (F) 2"="reset? (F) 2", "manual control 2"="manual control 2", "Gains Z"="Gains Z", "setpoint weighting 3"="setpoint weighting 3", "output range 3"="output range 3", "reset? (F) 3"="reset? (F) 3", "manual control 3"="manual control 3") -> ("FPGA VI Reference Out"=w54:refnum<k20>, "error out"=w52:errorcluster, "actions 2"=→"actions 2":T9, "output 2"=→"output 2":sgl, "error 2"=→"error 2":sgl, "actions 3"=→"actions 3":T9, "output 3"=→"output 3":sgl, "error 3"=→"error 3":sgl)
    n143 = Or(x="stop", y=w52) -> (x .or. y?=w58:bool)
    n144 = in-place {
      in-place-border: [w288] -> w59
      in-place-border: w58 -> [w286]
      n145 = in-place-dvr #6(w154) -> (w289:bool, w287:errorcluster)
      n146 = Compound Arithmetic op=OR(w286, w289, w287) -> (w288:bool)
      n147 = in-place-dvr #6(w288) -> ()  [unwired: 2 out]
    }
    n148 = Wait (ms)(milliseconds to wait=u32 33) -> ()  [unwired: 1 out]
  }
  n149 = while {
    tunnel: [w360] -> _
    tunnel: w2 -> [w359]
    tunnel: w13 -> [w341]
    tunnel: w10 -> [w356]
    tunnel: w5 -> [w358]
    tunnel: [w346] -> w9
    tunnel: w12 -> [w342]
    stop <- w357 stop-if-true
    w333 = 0  # Waveform recording stream index
    # "The example interleaves 4 channels of data into one stream."
    # "Wait for the transfer to complete.  This will report overflows if they occur during the transfer."
    # "Configure the AI stream for a finite recording and start"
    # "Configure the input channel and trigger"
    # "Analog Input"
    n150 = call "Volts to Codes.vi"("range (Vpp)"=w341, "Number of Bits"=i16 16, "Volts In"="Data Trigger Level (V)") -> ("ADC Codes Out"=w343:i16)  [unwired: 8 in]
    n151 = Bundle By Name(cluster=T10 {"level"=0, "trigger when"=enum."Trigger Above"} ("Trigger Configuration"), "level"=w343, "trigger when"="Data Trigger When") -> (w332:T10)
    n152 = xnode "Read/Write Control"("FPGA VI Reference In"=w359, "error in"=w358, "Trigger Type"="Trigger Type", "Trigger Configuration"=w332) -> ("FPGA VI Reference Out"=w337:refnum<k20>, "error out"=w336:errorcluster)
    n153 = call <instrlib>:"Clear Stream.vi"("error in (no error)"=w336, "stream index"=w333, "refnum in"=w337) -> ("error out"=w335:errorcluster, "refnum out"=w334:refnum<k20>)  [unwired: 7 in]
    n154 = Multiply(x="Record Size", y=u16 4) -> (x*y=w338:u16)
    n155 = call-poly <instrlib>:"Start Stream.vi"("error in (no error)"=w335, "num samples"=w338, "stream index"=w333, "refnum in"=w334) -> ("error out"=w351:errorcluster, "refnum out"=w349:refnum<k20>)  [unwired: 6 in]
    n156 = call-poly <instrlib>:"Wait.vi"("error in (no error)"=w351, "stream index"=w333, "refnum in"=w349) -> ("error out"=w347:errorcluster, "samples transferred"=w350:u64, "refnum out"=w348:refnum<k20>)  [unwired: 5 in, 1 out]
    n157 = xnode "Invoke Method"("FPGA VI Reference In"=w348, "error in"=w347, "Number of Elements"=w350) -> ("FPGA VI Reference Out"=w360:refnum<k20>, "error out"=w346:errorcluster, "Data"=w354:i16[])  [unwired: 1 in, 1 out]
    n158 = call "Scale Acquired Data NI 5783.vi"("range (V)"=w341, "Sample Rate"=w342, "Number of Bits"=i16 16, "Data In"=w354) -> ("Data"=→"AI":waveform(dbl)[])  [unwired: 7 in]
    n159 = in-place {
      in-place-border: [w363] -> w357
      in-place-border: w346 -> [w365]
      n160 = in-place-dvr #7(w356) -> (w364:bool, w362:errorcluster)
      n161 = Compound Arithmetic op=OR(w365, w364, w362) -> (w363:bool)
      n162 = in-place-dvr #7(w363) -> ()  [unwired: 2 out]
    }
    n163 = Wait (ms)(milliseconds to wait=u32 100) -> ()  [unwired: 1 out]
  }
  n164 = Merge Errors(w9, w8) -> (w11:errorcluster)
  n165 = xnode "Read/Write Control"("FPGA VI Reference In"=w17, "error in"=w11, "stream.request state 2"=3) -> ("FPGA VI Reference Out"=w14:refnum<k20>, "error out"=w16:errorcluster)
  n166 = xnode "Close FPGA VI Reference"("FPGA VI Reference In"=w14, "error in"=w16) -> ("error out"=w24:errorcluster)
  n167 = call <vilib>:"Simple Error Handler.vi"("error in (no error)"=w24) -> ("error out"=→"Error Out":errorcluster)  [unwired: 4 in, 4 out]
